vi "Set Lamp Power.vi"(8 "error in (no error)":errorcluster, 10 "Level":u8 max=150 step=1, 11 "Neph in":refnum<class "Nephelometer.lvclass">) -> (0 "error out":errorcluster, 3 "Neph out":refnum<class "Nephelometer.lvclass">)   [LabVIEW 2014, in "Nephelometer.lvclass"]
uses:
  Nephelometer.lvclass
  Reusable/Session APIs/Serial/Serial Session.lvclass
  Nephelometer.lvclass/Nephelometer.ctl
  Accessors/Read Session Handle.vi
  <userlib>/_Session Fwk/Session - Root.lvclass
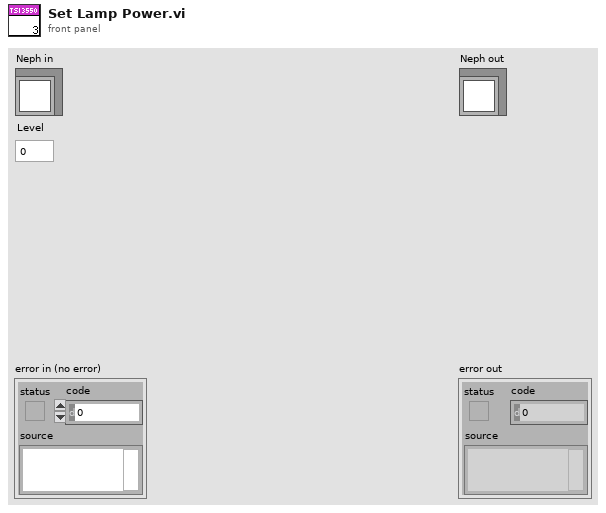
[diagram p1: front panel]
types:
  T1 = typedef "Session - Root.lvclass/Session Handle.ctl" = refnum<data-value>
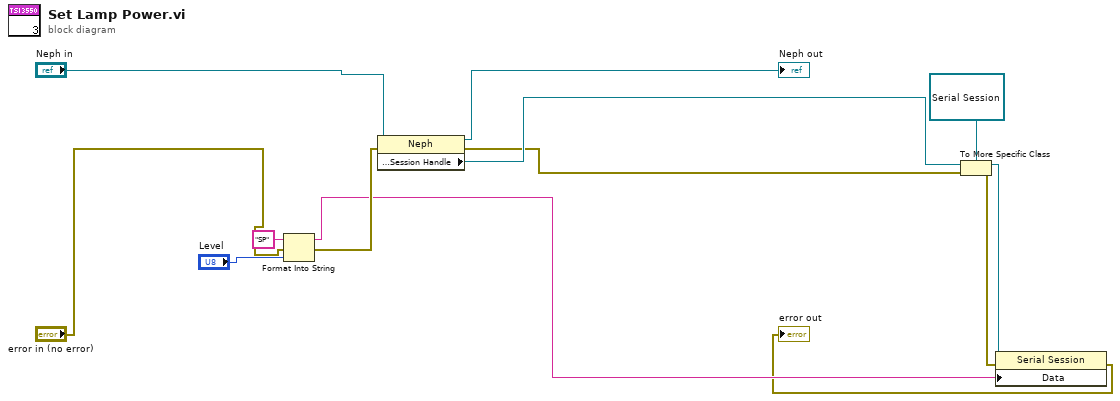
[diagram p0: block diagram]
diagram:
  n1 = Format Into String(initial string="SP", error in="error in (no error)", "Level") -> (resulting string=w4:string, error out=w8:errorcluster)  [unwired: 1 in]
  n2 = property class="Neph"(reference="Neph in", error in=w8) -> (reference out=→"Neph out":refnum<class "Nephelometer.lvclass">, error out=w2:errorcluster, "Accessors:Session Handle"=w3:T1)
  n3 = To More Specific Class(target class=refnum<data-value> refnum ("Session Handle"), reference=w3, error in=w2) -> (specific class reference=w6:refnum<data-value>, error out=w5:errorcluster)
  n4 = property class="Serial Session"(reference=w6, error in=w5, "Data"=w4) -> (error out=→"error out":errorcluster)  [unwired: 1 out]
